vi "MHM Read Ports.vi"(8 "error in (no error)":errorcluster, 11 "ulMHMHandle":u32) -> (0 "error out":errorcluster, 2 "pulPorts":u32, 3 "function return":u32)   [LabVIEW 2019, in "MHM_1SL_interface.lvlib"]
uses:
  MHM_1SL_interface.lvlib
  lib/MHM_1SL_interface.dll
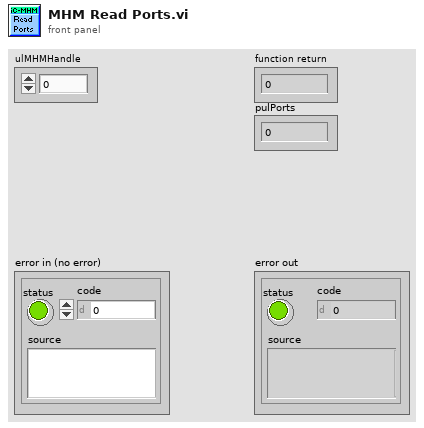
[diagram p1: front panel]
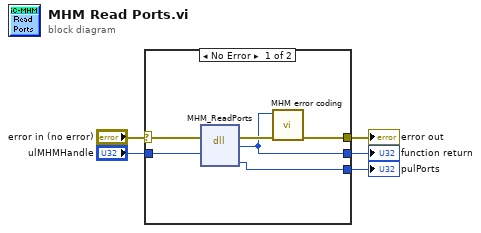
[diagram p0: block diagram]
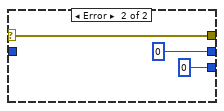
[diagram p2: hidden frame]
diagram:
  n1 = case shown="No Error" "error in (no error)" {
    selector: "error in (no error)" -> [w11 w14]
    tunnel: "ulMHMHandle" -> [w9 _]
    tunnel: [w8 w14] -> w3
    tunnel: [w7 u32 0 ("return type")] -> w2
    tunnel: [w6 u32 0 ("pulValid")] -> w1
    frame No Error {
      n2 = dll-call lib="C:/workspace/project/scancon/MHM_1SL_interface_4.4.0/lv_interface/lib/MHM_1SL_interface.dll" fn="MHM_ReadPorts"(error in=w11, "ulMHMHandle"=w9) -> (error out=w10:errorcluster, "return type"=w7:u32, "pulPorts"=w6:u32)  [unwired: 4 in, 1 out]
      n3 = call "MHM error coding.vi"("error in (no error)"=w10, "function return in"=w7) -> ("error out"=w8:errorcluster)  [unwired: 9 in]
    }
    frame Error {
    }
  }
  "function return" <- w2
  "pulPorts" <- w1
  "error out" <- w3
